vi "time_unit_conversion_sec_to_scan.vi"(1 "time duration (s)":dbl caption="时间长度 (s)") -> (0 "time duration (scan)":i64 caption="时间长度 (scan)")   [LabVIEW 2015]
uses:
  globals/global_configuration_options.vi
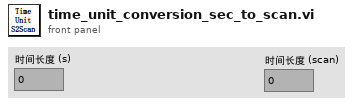
[diagram p1: front panel]
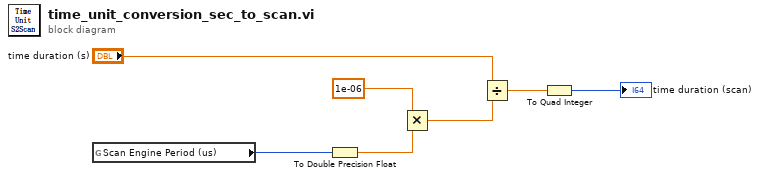
[diagram p0: block diagram]
diagram:
  n1 = global read "global_configuration_options.vi" "Scan Engine Period (us)"() -> (w1:u32)
  n2 = To Double Precision Float(number=w1) -> (double precision float=w3:dbl)
  n3 = Multiply(x=1e-06 ("y"), y=w3) -> (x*y=w5:dbl)
  n4 = Divide(x="time duration (s)", y=w5) -> (x/y=w6:dbl)
  n5 = To Quad Integer(1:w6) -> (0:→"time duration (scan)":i64)
